vi "esp_gpib_send_ASCII.vi"(4 "mode (0)":i16, 7 "ASCII Cmd":string="tb", 8 "Delay In":u16, 9 "error in":errorcluster, 10 "Status In":i32, 11 "Port In":i32) -> (0 "Delay Out":u16, 1 "error out":errorcluster, 2 "Status Out":i32, 3 "Port Out":i32, 6 "StringOut":string="tb\r")   [LabVIEW 2015]
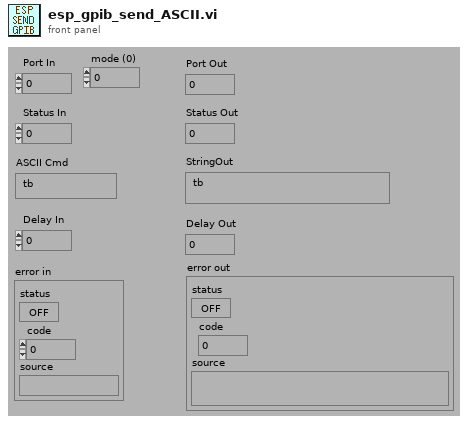
[diagram p1: front panel]
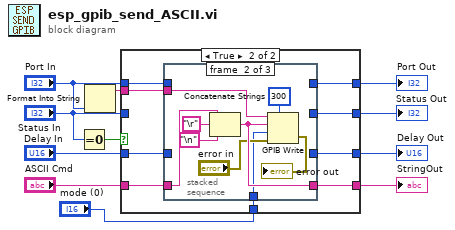
[diagram p0: block diagram]
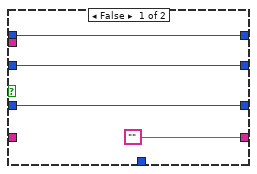
[diagram p2: hidden frame]
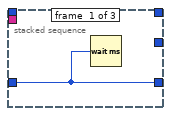
[diagram p3: hidden frame]
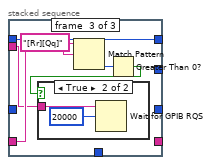
[diagram p4: hidden frame]
diagram:
  n1 = Equal To 0?(x="Status In") -> (x = 0?=w11:bool)
  n2 = Format Into String("Port In") -> (resulting string=w2:string)  [unwired: 3 in, 1 out]
  n3 = case shown="True" w11 {
    tunnel: [w15 w23] -> w10
    tunnel: "Delay In" -> [w15 w24]
    tunnel: "Status In" -> [w14 _]
    tunnel: [w14 w19] -> w7
    tunnel: "ASCII Cmd" -> [_ w22]
    tunnel: "Port In" -> [w12 w21]
    tunnel: ["" w20] -> w5
    tunnel: [w12 w17] -> w4
    tunnel: w2 -> [_ w18]
    tunnel: "mode (0)" -> [_ w16]
    frame False {
    }
    frame True {
      n4 = stacked-sequence {
        tunnel: w24 -> [w25 _ _]
        tunnel: [w25 _ _] -> w23
        tunnel: w22 -> [_ w35 w39]
        tunnel: w21 -> [_ _ w36]
        tunnel: [_ w32 _] -> w20
        tunnel: [_ 0 _] -> w19
        tunnel: w18 -> [_ w30 w37]
        tunnel: [_ _ w36] -> w17
        tunnel: w16 -> [_ w26 _]
        frame #0 {
          n5 = Wait (ms)(milliseconds to wait=w25) -> ()  [unwired: 1 out]
        }
        frame #1 {
          n6 = Concatenate Strings(w35, "\r", "\n") -> (w32:string)
          n7 = GPIB Write(0:w30, 1:w32, 2:w26, 3:"error in", 4:300 ("timeout ms (488.2 global)")) -> (6:→"error out":errorcluster)  [unwired: 1 out]
        }
        frame #2 {
          n8 = Match Pattern(string=w39, regular expression="[Rr][Qq]") -> (offset past match=w41:i32)  [unwired: 1 in, 3 out]
          n9 = Greater Than 0?(x=w41) -> (x > 0?=w38:bool)
          n10 = case shown="True" w38 {
            tunnel: w37 -> [_ w42]
            frame False {
            }
            frame True {
              n11 = Wait for GPIB RQS(3:20000 ("timeout ms (488.2 global)"), 4:w42) -> ()  [unwired: 1 in, 2 out]
            }
          }
        }
      }
    }
  }
  "Delay Out" <- w10
  "Status Out" <- w7
  "StringOut" <- w5
  "Port Out" <- w4
